vi "Write Runtime Data.vi"(7 "Section Name":string="PluginSpecific", 8 "error in":errorcluster, 10 "Runtime Data In":T1, 11 "Config File Data In":T2(array[cluster])) -> (0 "error out":errorcluster, 2 "Runtime Data Out":T1, 3 "Config Data Out":T2(array[cluster]))   [LabVIEW 2020, in "GUCalibration2.lvlib"]
uses:
  GUCalibration2.lvlib
  Controls/Config Data Type.ctl
  Utilities/Write Key I32.vi
  Utilities/Write Key Boolean.vi
  Utilities/Write Key String.vi
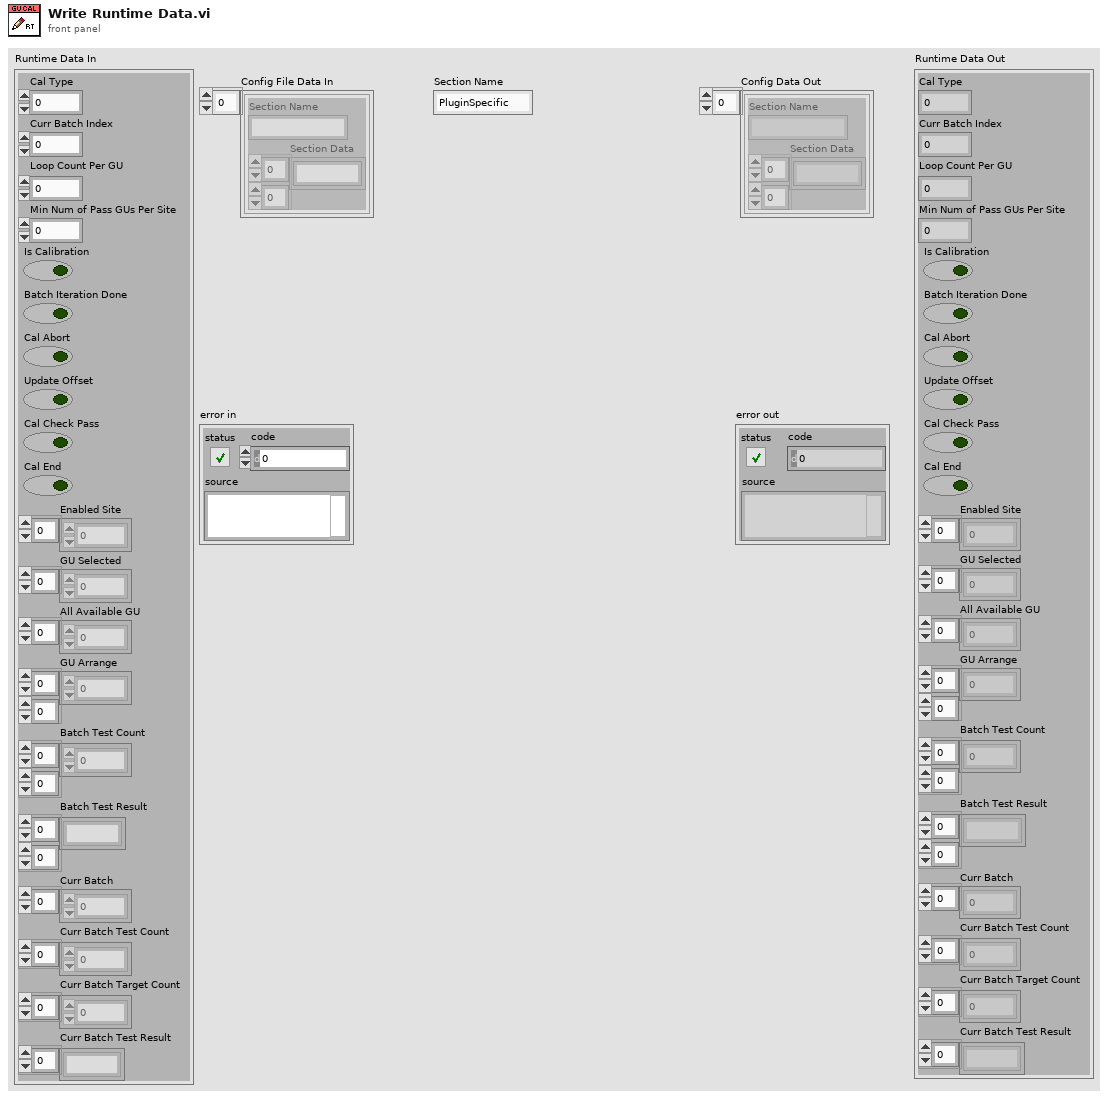
[diagram p1: front panel]
types:
  T1 = typedef "GUCalibration2.lvlib/Config Data Type.ctl" = cluster{"Cal Type":i32, "Curr Batch Index":i32, "Loop Count Per GU":i32, "Min Num of Pass GUs Per Site":i32, "Is Calibration":bool, "Batch Iteration Done":bool, "Cal Abort":bool, "Update Offset":bool, "Cal Check Pass":bool, "Cal End":bool, "Enabled Site":i32[], "GU Selected":i32[], "All Available GU":i32[], "GU Arrange":i32[][], "Batch Test Count":i32[][], "Batch Test Result":string[][], "Curr Batch":i32[], "Curr Batch Test Count":i32[], "Curr Batch Target Count":i32[], "Curr Batch Test Result":string[]}
  T2 = cluster{"Section Name":string, "Section Data":string[][]}[]
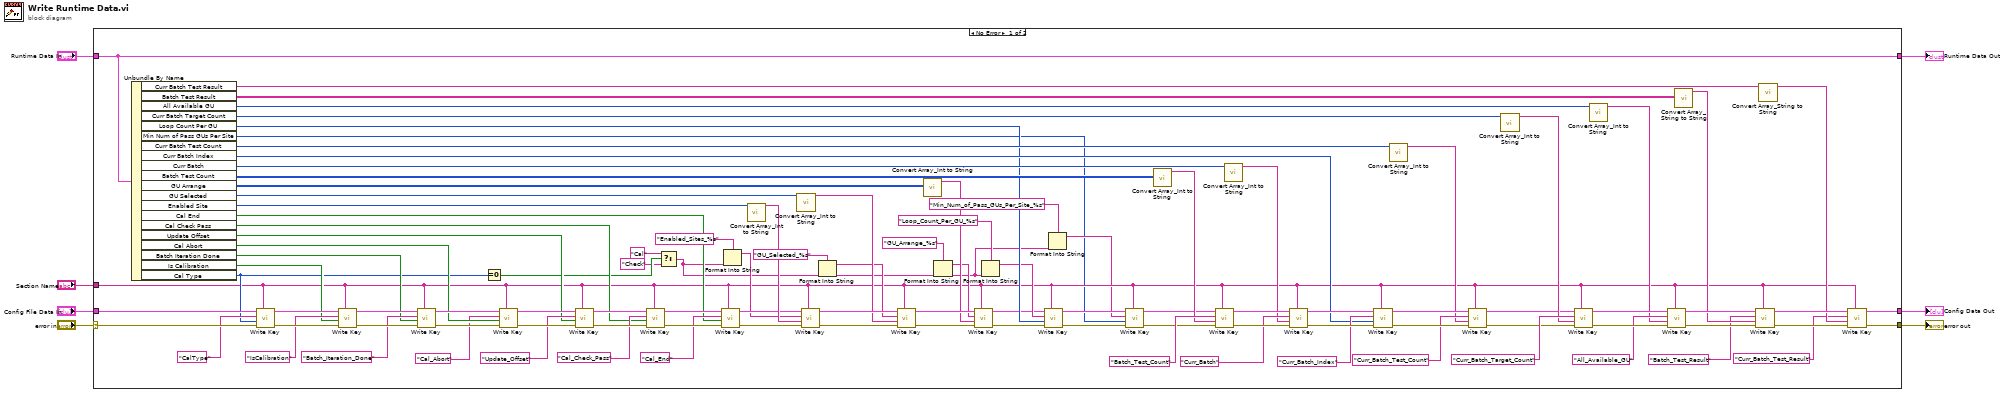
[diagram p0: block diagram]
diagram:
  n1 = case shown="No Error" "error in" {
    selector: "error in" -> [w95 w112]
    tunnel: "Config File Data In" -> [w96 w111]
    tunnel: "Section Name" -> [w12 _]
    tunnel: [w59 w112] -> w5
    tunnel: [w79 _] -> w4
    tunnel: [w58 w111] -> w2
    tunnel: "Runtime Data In" -> [w79 _]
    frame No Error {
      n2 = Unbundle By Name(w79) -> ("Curr Batch Test Result"=w55:string[], "Batch Test Result"=w57:string[][], "All Available GU"=w65:i32[], "Curr Batch Target Count"=w78:i32[], "Loop Count Per GU"=w80:i32, "Min Num of Pass GUs Per Site"=w8:i32, "Curr Batch Test Count"=w82:i32[], "Curr Batch Index"=w83:i32, "Curr Batch"=w85:i32[], "Batch Test Count"=w87:i32[][], "GU Arrange"=w89:i32[][], "GU Selected"=w91:i32[], "Enabled Site"=w93:i32[], "Cal End"=w33:bool, "Cal Check Pass"=w39:bool, "Update Offset"=w41:bool, "Cal Abort"=w48:bool, "Batch Iteration Done"=w51:bool, "Is Calibration"=w69:bool, "Cal Type"=w24:i32)
      n3 = call-poly "Write Key.vi"("Section Name"=w12, "error in (no error)"=w95, "Key Value"=w24, "Key Name"="CalType" ("Section Name"), "Config Data"=w96) -> ("error out"=w76:errorcluster, "Config Data dup"=w77:T2)  [unwired: 5 in]
      n4 = call-poly "Write Key.vi"("Section Name"=w12, "error in (no error)"=w76, "Key Value"=w69, "Key Name"="IsCalibration" ("Section Name"), "Config Data"=w77) -> ("error out"=w71:errorcluster, "Config Data dup"=w72:T2)  [unwired: 5 in]
      n5 = call-poly "Write Key.vi"("Section Name"=w12, "error in (no error)"=w71, "Key Value"=w51, "Key Name"="Batch_Iteration_Done" ("Section Name"), "Config Data"=w72) -> ("error out"=w49:errorcluster, "Config Data dup"=w50:T2)  [unwired: 5 in]
      n6 = Equal To 0?(x=w24) -> (x = 0?=w23:bool)
      n7 = call-poly "Write Key.vi"("Section Name"=w12, "error in (no error)"=w49, "Key Value"=w48, "Key Name"="Cal_Abort" ("Section Name"), "Config Data"=w50) -> ("error out"=w45:errorcluster, "Config Data dup"=w46:T2)  [unwired: 5 in]
      n8 = call-poly "Write Key.vi"("Section Name"=w12, "error in (no error)"=w45, "Key Value"=w41, "Key Name"="Update_Offset" ("Section Name"), "Config Data"=w46) -> ("error out"=w43:errorcluster, "Config Data dup"=w44:T2)  [unwired: 5 in]
      n9 = call-poly "Write Key.vi"("Section Name"=w12, "error in (no error)"=w43, "Key Value"=w39, "Key Name"="Cal_Check_Pass" ("Section Name"), "Config Data"=w44) -> ("error out"=w37:errorcluster, "Config Data dup"=w38:T2)  [unwired: 5 in]
      n10 = Select(t="Cal" ("Section Name"), s=w23, f="Check" ("Section Name")) -> (s? t:f=w10:string)
      n11 = call-poly "Write Key.vi"("Section Name"=w12, "error in (no error)"=w37, "Key Value"=w33, "Key Name"="Cal_End" ("Section Name"), "Config Data"=w38) -> ("error out"=w35:errorcluster, "Config Data dup"=w36:T2)  [unwired: 5 in]
      n12 = Format Into String(format string="Enabled_Sites_%s" ("Section Name"), w10) -> (resulting string=w25:string)  [unwired: 2 in, 1 out]
      n13 = call "Convert Array_Int to String.vi"("Data 1"=w93) -> ("String Out"=w92:string)  [unwired: 10 in]
      n14 = call "Convert Array_Int to String.vi"("Data 1"=w91) -> ("String Out"=w90:string)  [unwired: 10 in]
      n15 = call-poly "Write Key.vi"("Section Name"=w12, "error in (no error)"=w35, "Key Value"=w92, "Key Name"=w25, "Config Data"=w36) -> ("error out"=w110:errorcluster, "Config Data dup"=w109:T2)  [unwired: 5 in]
      n16 = Format Into String(format string="GU_Selected_%s" ("Section Name"), w10) -> (resulting string=w30:string)  [unwired: 2 in, 1 out]
      n17 = call-poly "Write Key.vi"("Section Name"=w12, "error in (no error)"=w110, "Key Value"=w90, "Key Name"=w30, "Config Data"=w109) -> ("error out"=w107:errorcluster, "Config Data dup"=w108:T2)  [unwired: 5 in]
      n18 = call "Convert Array_Int to String.vi"("Data 2"=w89) -> ("String Out"=w88:string)  [unwired: 10 in]
      n19 = Format Into String(format string="GU_Arrange_%s" ("Section Name"), w10) -> (resulting string=w28:string)  [unwired: 2 in, 1 out]
      n20 = call-poly "Write Key.vi"("Section Name"=w12, "error in (no error)"=w107, "Key Value"=w88, "Key Name"=w28, "Config Data"=w108) -> ("error out"=w19:errorcluster, "Config Data dup"=w20:T2)  [unwired: 5 in]
      n21 = Format Into String(format string="Loop_Count_Per_GU_%s" ("Section Name"), w10) -> (resulting string=w27:string)  [unwired: 2 in, 1 out]
      n22 = call-poly "Write Key.vi"("Section Name"=w12, "error in (no error)"=w19, "Key Value"=w80, "Key Name"=w27, "Config Data"=w20) -> ("error out"=w15:errorcluster, "Config Data dup"=w16:T2)  [unwired: 5 in]
      n23 = Format Into String(format string="Min_Num_of_Pass_GUs_Per_Site_%s" ("Section Name"), w10) -> (resulting string=w9:string)  [unwired: 2 in, 1 out]
      n24 = call-poly "Write Key.vi"("Section Name"=w12, "error in (no error)"=w15, "Key Value"=w8, "Key Name"=w9, "Config Data"=w16) -> ("error out"=w13:errorcluster, "Config Data dup"=w14:T2)  [unwired: 5 in]
      n25 = call "Convert Array_Int to String.vi"("Data 2"=w87) -> ("String Out"=w86:string)  [unwired: 10 in]
      n26 = call-poly "Write Key.vi"("Section Name"=w12, "error in (no error)"=w13, "Key Value"=w86, "Key Name"="Batch_Test_Count" ("Section Name"), "Config Data"=w14) -> ("error out"=w104:errorcluster, "Config Data dup"=w105:T2)  [unwired: 5 in]
      n27 = call "Convert Array_Int to String.vi"("Data 1"=w85) -> ("String Out"=w84:string)  [unwired: 10 in]
      n28 = call-poly "Write Key.vi"("Section Name"=w12, "error in (no error)"=w104, "Key Value"=w84, "Key Name"="Curr_Batch" ("Section Name"), "Config Data"=w105) -> ("error out"=w101:errorcluster, "Config Data dup"=w102:T2)  [unwired: 5 in]
      n29 = call-poly "Write Key.vi"("Section Name"=w12, "error in (no error)"=w101, "Key Value"=w83, "Key Name"="Curr_Batch_Index" ("Section Name"), "Config Data"=w102) -> ("error out"=w98:errorcluster, "Config Data dup"=w99:T2)  [unwired: 5 in]
      n30 = call "Convert Array_Int to String.vi"("Data 1"=w82) -> ("String Out"=w81:string)  [unwired: 10 in]
      n31 = call-poly "Write Key.vi"("Section Name"=w12, "error in (no error)"=w98, "Key Value"=w81, "Key Name"="Curr_Batch_Test_Count" ("Section Name"), "Config Data"=w99) -> ("error out"=w17:errorcluster, "Config Data dup"=w18:T2)  [unwired: 5 in]
      n32 = call "Convert Array_Int to String.vi"("Data 1"=w78) -> ("String Out"=w73:string)  [unwired: 10 in]
      n33 = call-poly "Write Key.vi"("Section Name"=w12, "error in (no error)"=w17, "Key Value"=w73, "Key Name"="Curr_Batch_Target_Count" ("Section Name"), "Config Data"=w18) -> ("error out"=w67:errorcluster, "Config Data dup"=w68:T2)  [unwired: 5 in]
      n34 = call "Convert Array_Int to String.vi"("Data 1"=w65) -> ("String Out"=w64:string)  [unwired: 10 in]
      n35 = call-poly "Write Key.vi"("Section Name"=w12, "error in (no error)"=w67, "Key Value"=w64, "Key Name"="All_Available_GU" ("Section Name"), "Config Data"=w68) -> ("error out"=w62:errorcluster, "Config Data dup"=w63:T2)  [unwired: 5 in]
      n36 = call "Convert Array_String to String.vi"("Data 2"=w57) -> ("String Out"=w56:string)  [unwired: 10 in]
      n37 = call-poly "Write Key.vi"("Section Name"=w12, "error in (no error)"=w62, "Key Value"=w56, "Key Name"="Batch_Test_Result" ("Section Name"), "Config Data"=w63) -> ("error out"=w60:errorcluster, "Config Data dup"=w61:T2)  [unwired: 5 in]
      n38 = call "Convert Array_String to String.vi"("Data 1"=w55) -> ("String Out"=w54:string)  [unwired: 10 in]
      n39 = call-poly "Write Key.vi"("Section Name"=w12, "error in (no error)"=w60, "Key Value"=w54, "Key Name"="Curr_Batch_Test_Result" ("Section Name"), "Config Data"=w61) -> ("error out"=w59:errorcluster, "Config Data dup"=w58:T2)  [unwired: 5 in]
    }
    frame Error {
    }
  }
  "error out" <- w5
  "Runtime Data Out" <- w4
  "Config Data Out" <- w2
